vi "New Library.vi"(8 "error in (no error)":errorcluster) -> (0 "error out":errorcluster, 3 "Library:Create":refnum<vi>)   [LabVIEW 2017, in "WebServiceImporter.lvlib" / "VI Generator.lvlib"]
uses:
  <vilib>/Platform/WebService/VI Generator/VI Generator.lvlib
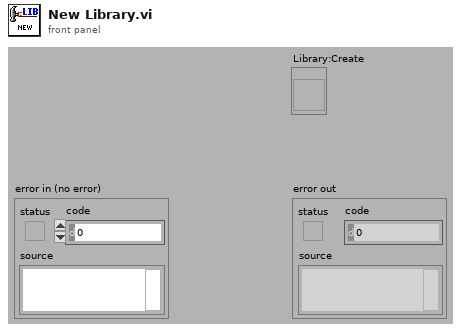
[diagram p1: front panel]
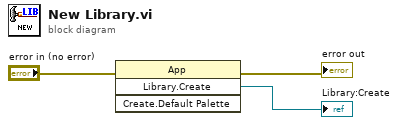
[diagram p0: block diagram]
diagram:
  n1 = invoke class="App" method="Library.Create"(error in="error in (no error)") -> (error out=→"error out":errorcluster, "Create Library"=→"Library:Create":refnum<vi>)  [unwired: 3 in, 2 out]
